vi "GF_addToLog.vi"(2 "error in":errorcluster, 3 "Value":i32, 4 "Key Name":string, 5 "Current String":string) -> (0 "error out":errorcluster, 1 "concatenated string":string)   [LabVIEW 2016]
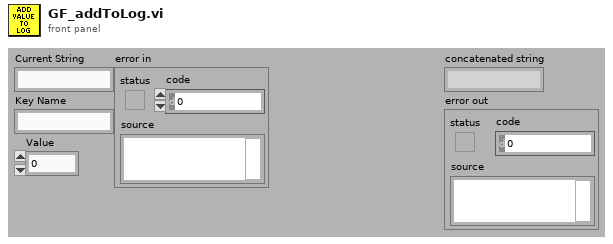
[diagram p1: front panel]
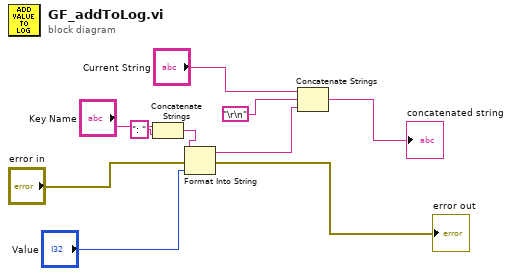
[diagram p0: block diagram]
diagram:
  n1 = Concatenate Strings("Key Name", ": " ("string")) -> (w2:string)
  n2 = Format Into String(initial string=w2, error in="error in", "Value") -> (resulting string=w6:string, error out=→"error out":errorcluster)  [unwired: 1 in]
  n3 = Concatenate Strings("Current String", "\r\n", w6) -> (→"concatenated string":string)
